vi "RaiseForTimeController.vi"(9 "Command Timing":cluster{"Start Time (ms)":u32, "Iterations":i32}, 10 "Speed":dbl, 11 "Time":dbl) -> (0 "Delay":dbl, 1 "Demand1":dbl, 2 "DemandType":T2(ring), 3 "Control Mode":T1 items=["PercentOutput"=0, "Position"=1, "Velocity"=2, "Current"=3, "Follower"=5, "MotionProfile"=6, "MotionMagic"=7, "MotionProfileArc"=10, "Disabled"=15], 4 "Done":bool, 5 "SpeedOut":dbl)   [LabVIEW 2018]
uses:
  <vilib>/Rock Robotics/WPI/ThirdParty/Phoenix-LabVIEW/Motor Controller/Controls/CTRE_Phoenix_MotorControl_ControlMode.ctl
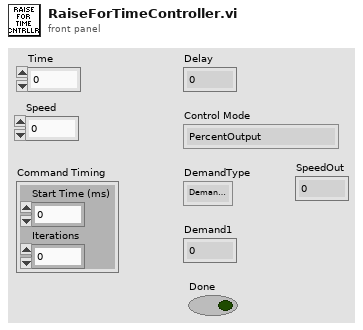
[diagram p1: front panel]
types:
  T1 = typedef "CTRE_Phoenix_MotorControl_ControlMode.ctl" = u16
  T2 = enum16{"DemandType_Neutral", "DemandType_AuxPID", "DemandType_ArbitraryFeedForward"}
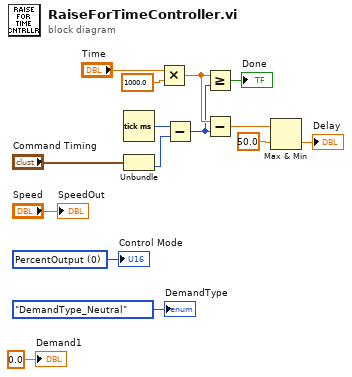
[diagram p0: block diagram]
diagram:
  w13 = T1 0 items=["PercentOutput"=0, "Position"=1, "Velocity"=2, "Current"=3, "Follower"=5, "MotionProfile"=6, "MotionMagic"=7, "MotionProfileArc"=10, "Disabled"=15] ("Control Mode")
  n1 = Tick Count (ms)() -> (millisecond timer value=w2:u32)
  n2 = Unbundle("Command Timing") -> ("Iterations"=w6:i32)  [unwired: 1 out]
  n3 = Multiply(x="Time", y=1000.0) -> (x*y=w7:dbl)
  n4 = Subtract(x=w2, y=w6) -> (x-y=w3:u32)
  n5 = Greater Or Equal?(x=w7, y=w3) -> (x >= y?=→"Done":bool)
  n6 = Subtract(x=w7, y=w3) -> (x-y=w5:dbl)
  n7 = Max & Min(x=w5, y=50.0) -> (min(x,y)=→"Delay":dbl)  [unwired: 1 out]
  "Demand1" <- 0.0 ("Demand1")
  "DemandType" <- T2."DemandType_Neutral" ("DemandType")
  "Control Mode" <- w13
  "SpeedOut" <- "Speed"
